vi "ExSubCreateData.vi"(2 "error in (no error)":errorcluster, 3 "File and Display Name":string, 4 "Pulser Handle":u32, 5 "Camera Handle":u32) -> (0 "error out":errorcluster, 1 "Handles Out":T1)   [LabVIEW 2010]
panel:
  # "ExSubCreateData:\nThis is a SubVI that creates image \nobjects and returns the handles bundled in a cluster \nthat includes a pulser and camera handle"
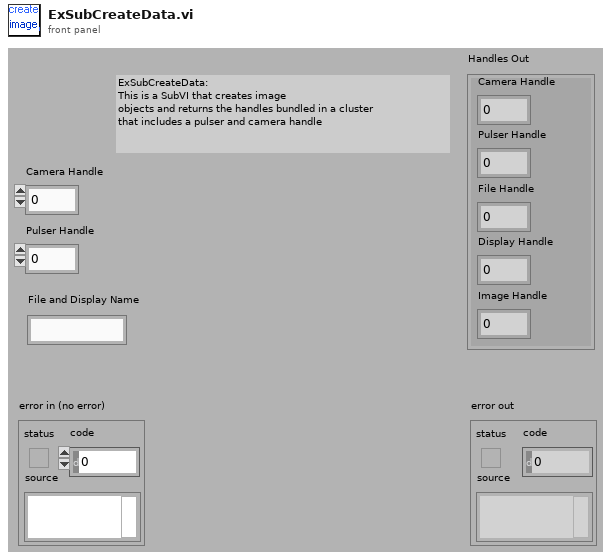
[diagram p1: front panel]
types:
  T1 = cluster{"Camera Handle":u32, "Pulser Handle":u32, "File Handle":u32, "Display Handle":u32, "Image Handle":u32}
  T2 = cluster{"Camera Handle":u32, "Pulser Handle":u32, i32, i32, "Image Handle":u32}
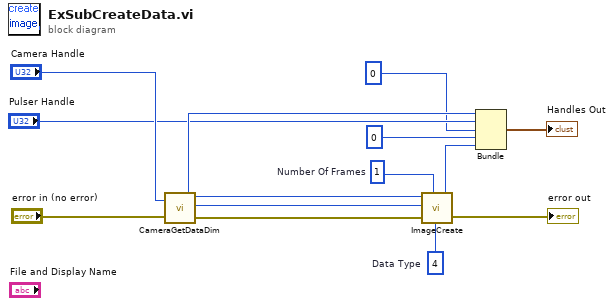
[diagram p0: block diagram]
diagram:
  w7 = u32 1  # Number Of Frames
  w8 = u32 4  # Data Type
  n1 = call <userlib>:"CameraGetDataDim.vi"("Camera Handle"="Camera Handle", "error in"="error in (no error)") -> ("Camera Handle"=w11:u32, "Xdim"=w3:u32, "Ydim"=w2:u32, "error out"=w14:errorcluster)
  n2 = call <userlib>:"ImageCreate.vi"("X dimension"=w3, "Y dimension"=w2, "Data Type"=w8, "error in"=w14, "Number Of Frames"=w7) -> ("Image Handle"=w9:u32, "error out"=→"error out":errorcluster)
  n3 = Bundle("Camera Handle"=w11, "Pulser Handle"="Pulser Handle", 0, 0, "Image Handle"=w9) -> (→"Handles Out":T2)  [unwired: 1 in]
